vi "GULTON_STRING_FORMER_MRW.vi"(0 "ACTION":enum16{"READ", "INCREASE", "DECREASE", "SET"}(ring), 1 "PARAMETER":T1, 2 "ZONE":u8=1 min=1 max=8, 3 "INPUT VALUE":dbl format="%.3f") -> (5 "STRING OUT":string)   [LabVIEW 2010]
uses:
  Gulton_Channel.ctl
panel:
  in  "PARAMETER":u16(ring) items=["Setpoint Maximum", "Power Limit", "Limit Comparator Value", "DERIATIVE TERM SETTING", "RANGE MAXIMUM", "RANGE MINIMUM", "INTEGRAL TERM SETTING", "STATUS", "MEASURED VARIABLE", "PROPORTIONAL BAND SETTING", "SETPOINT", "DEVIATION", "POWER OUTPUT LEVEL"]
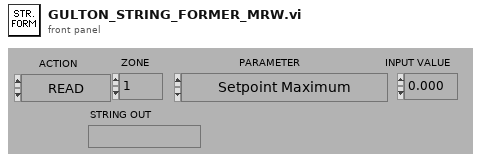
[diagram p1: front panel]
types:
  T1 = typedef "Gulton_Channel.ctl" = enum16{"Setpoint Maximum", "Power Limit", "Limit Comparator Value", "Derivative Term Setting", "Range Maximum", "Range Minimum", "Integral Term Setting", "Status", "MEASURED TEMPERATURE", "Proportional Band Setting", "SETPOINT", "Deviation", "POWER OUTPUT LEVEL"}
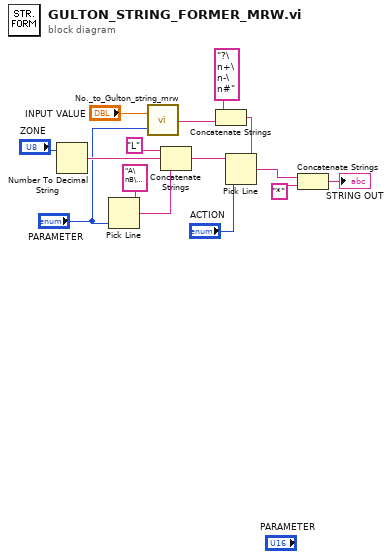
[diagram p0: block diagram]
diagram:
  n1 = Number To Decimal String(number="ZONE") -> (decimal integer string=w15:string)  [unwired: 1 in]
  n2 = Pick Line(multi-line string="A\nB\nC\nD\nG\nH\nI\nL\nM\nP\nS\nV\nW", line index="PARAMETER") -> (output string=w13:string)  [unwired: 1 in]
  n3 = call "No._to_Gulton_string_mrw.vi"("PARAMETER"="PARAMETER", "INPUT VALUE"="INPUT VALUE") -> ("OUTPUT STRING"=w3:string)  [unwired: 1 in]
  n4 = Concatenate Strings("L" ("S"), w15, w13) -> (w6:string)
  n5 = Concatenate Strings("?\n+\n-\n#", w3) -> (w8:string)
  n6 = Pick Line(string ("")=w6, multi-line string=w8, line index="ACTION") -> (output string=w7:string)
  n7 = Concatenate Strings(w7, "*") -> (→"STRING OUT":string)
